vi "CMD_BEEPER_CONTROL.vi"(0 "Input_Data":string[](array[string]), 5 "Error In":errorcluster) -> (12 "Validate CheckSum":bool, 13 "Command":u8[](array[numeric])=[5, 247, 4, 128, 255, 0, 0, 0, 0, 0, 0, 0, 0, 0] format="%x", 14 "Response":bool, 15 "Ack":bool, 16 "Command":bool, 17 "Add CheckSum":bool, 18 "Status":bool, 19 "Error Out":errorcluster)   [LabVIEW 2014]
panel:
  # "Flags"
  # "Beeper Control Command:"
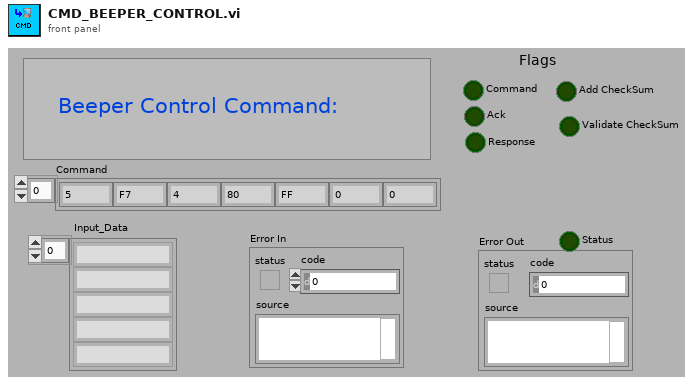
[diagram p1: front panel]
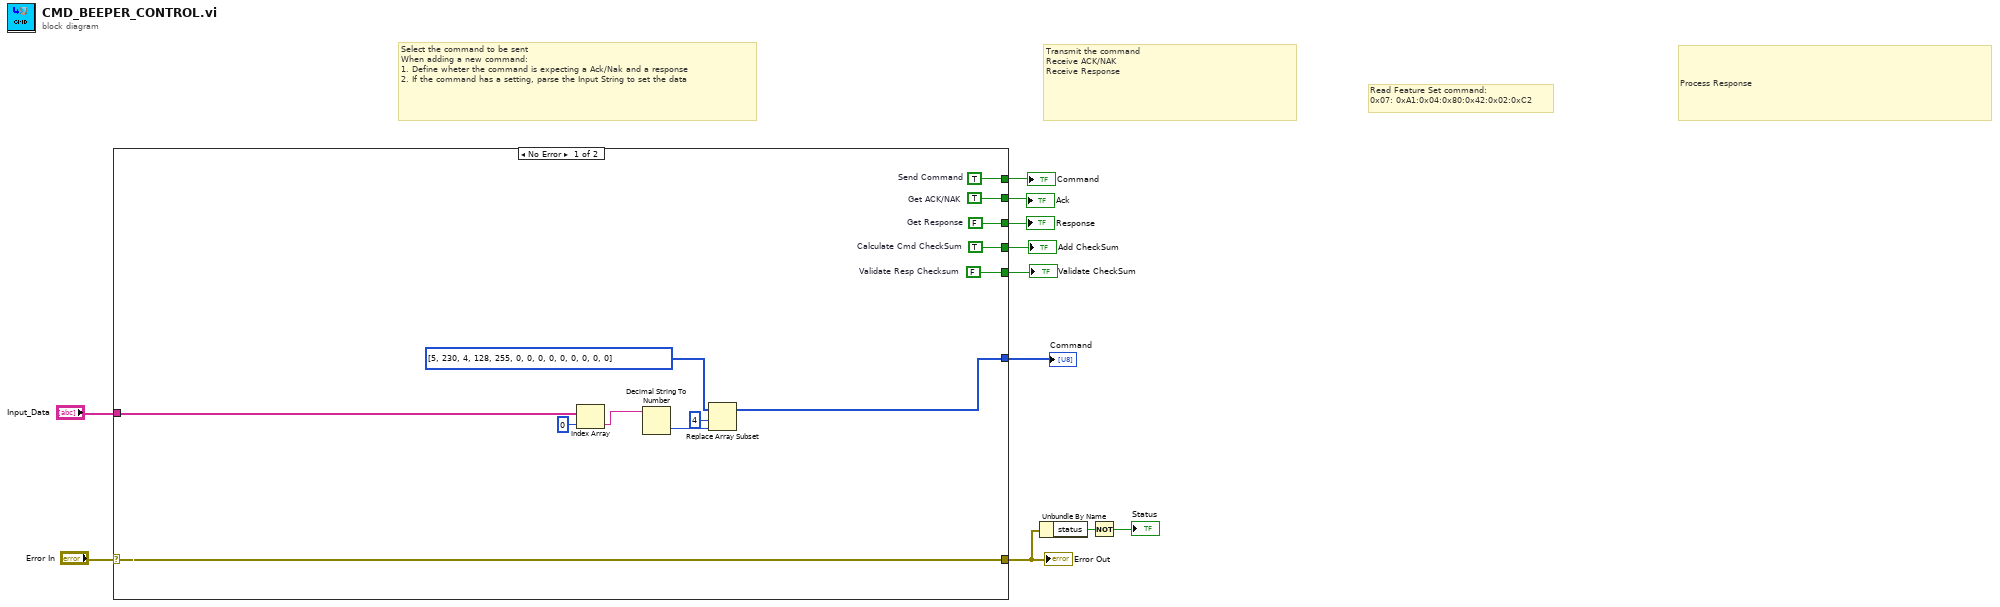
[diagram p0: block diagram]
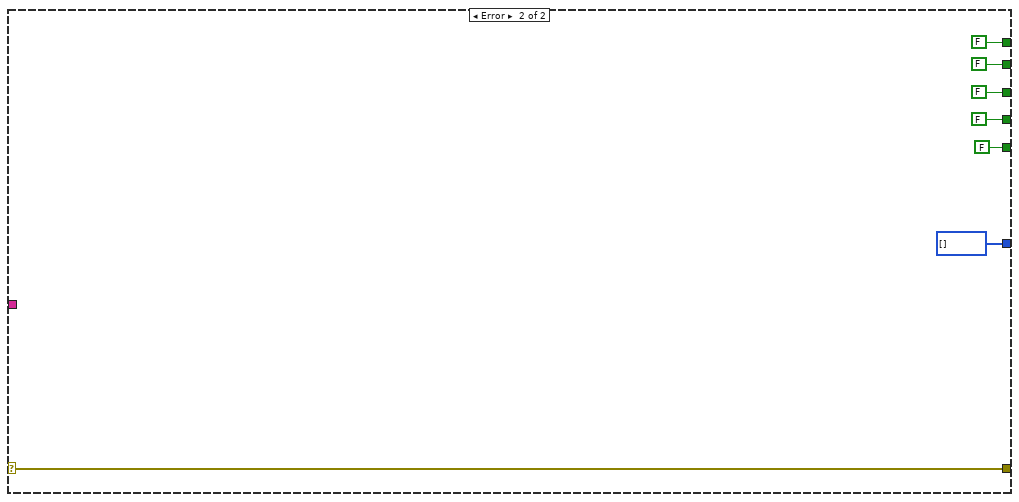
[diagram p2: hidden frame]
diagram:
  # "Read Feature Set command:\n0x07: 0xA1:0x04:0x80:0x42:0x02:0xC2"
  # "Process Response"
  # "Transmit the command\nReceive ACK/NAK\nReceive Response"
  # "Select the command to be sent\nWhen adding a new command:\n1. Define wheter the command is expecting a Ack/Nak and a response\n2. If the command has a setting, parse the Input String to set the data"
  n1 = case shown="No Error" "Error In" {
    selector: "Error In" -> [w20 w26]
    tunnel: [w24 FALSE ("Send Command")] -> w10
    tunnel: [w23 FALSE ("Get ACK/NAK")] -> w9
    tunnel: [w22 FALSE ("Get Response")] -> w8
    tunnel: [w21 FALSE ("Add CheckSum")] -> w7
    tunnel: [w12 u8[] []] -> w6
    tunnel: [w20 w26] -> w4
    tunnel: "Input_Data" -> [w15 _]
    tunnel: [w19 FALSE ("Validate Resp Checksum")] -> w1
    frame No Error {
      w19 = FALSE  # Validate Resp Checksum
      w21 = TRUE  # Calculate Cmd CheckSum
      w22 = FALSE  # Get Response
      w24 = TRUE  # Send Command
      w23 = TRUE  # Get ACK/NAK
      n2 = Index Array(array=w15, index=0) -> (element=w17:string)
      n3 = Decimal String To Number(string=w17) -> (number=w18:i32)  [unwired: 2 in, 1 out]
      n4 = Replace Array Subset(array=u8[] [5, 230, 4, 128, 255, 0, 0, 0, 0, 0, 0, 0, 0, 0], new element=w18, index=4) -> (w12:u8[])
    }
    frame Error {
    }
  }
  "Error Out" <- w4
  "Command" <- w10
  "Ack" <- w9
  "Response" <- w8
  "Add CheckSum" <- w7
  "Command" <- w6
  "Validate CheckSum" <- w1
  n5 = Unbundle By Name(w4) -> ("status"=w3:bool)
  n6 = Not(x=w3) -> (.not. x?=→"Status":bool)
